vi "MyTest_maximumSequence.vi"() -> ()   [LabVIEW 2018]
uses:
  VisionLibrariesXimea/xiLib/xiLIB_64bit/xiLIB/xiCamLib/xiLIB/Typedefs/xiLIB - PRM_Type.ctl
  VisionLibrariesXimea/xiLib/xiLIB_64bit/xiLIB/xiCamLib/xiLIB/Typedefs/xiLIB - PRM_Function.ctl
  VisionLibrariesXimea/xiLib/xiLIB_64bit/xiLIB/xiCamLib/xiCam/PRM/PRM/PRM_v2.ctl
  VisionLibrariesXimea/xiLib/xiLIB_64bit/xiLIB/xiCamLib/xiCam/PRM/ACQ_TIMING_MODE/ACQ_TIMING_MODE.ctl
  VisionLibrariesXimea/xiLib/xiLIB_64bit/xiLIB/xiCamLib/xiLIB/xiLIB - GetPRM_INFO.vi
  VisionLibrariesXimea/xiLib/xiLIB_64bit/xiLIB/xiCamLib/xiCam/Methods/xiCam - GetParam_Int32.vi
  VisionLibrariesXimea/xiLib/xiLIB_64bit/xiLIB/xiCamLib/xiCam/Methods/xiCam - GetParam_Float.vi
  VisionLibrariesXimea/xiLib/xiLIB_64bit/xiLIB/xiCamLib/xiCam/Methods/xiCam - GetParam_String.vi
panel:
  out "VI running":i32
  in  "input PRM":T1=enum."IMAGE_DATA_FORMAT_RGB32_ALPHA"
  out "Method":T2
  out "Type":T3
  out "output":variant
  in  "ask":bool
  out "error out":errorcluster
  in  "tot frame number":i32=10
  in  "stop":bool
  out "FFT":dbl[][](graph)
  out "Intensity Graph":u8[][](graph)
  in  "Exposure (us)":i32(slide) caption="Exposure (us) 1us - 1s steps of 1us" min=1 max=1000000 scale=0.9..5000.0
  in  "Height":i32 min=2 max=3424
  in  "Width":i32 min=32 max=4704
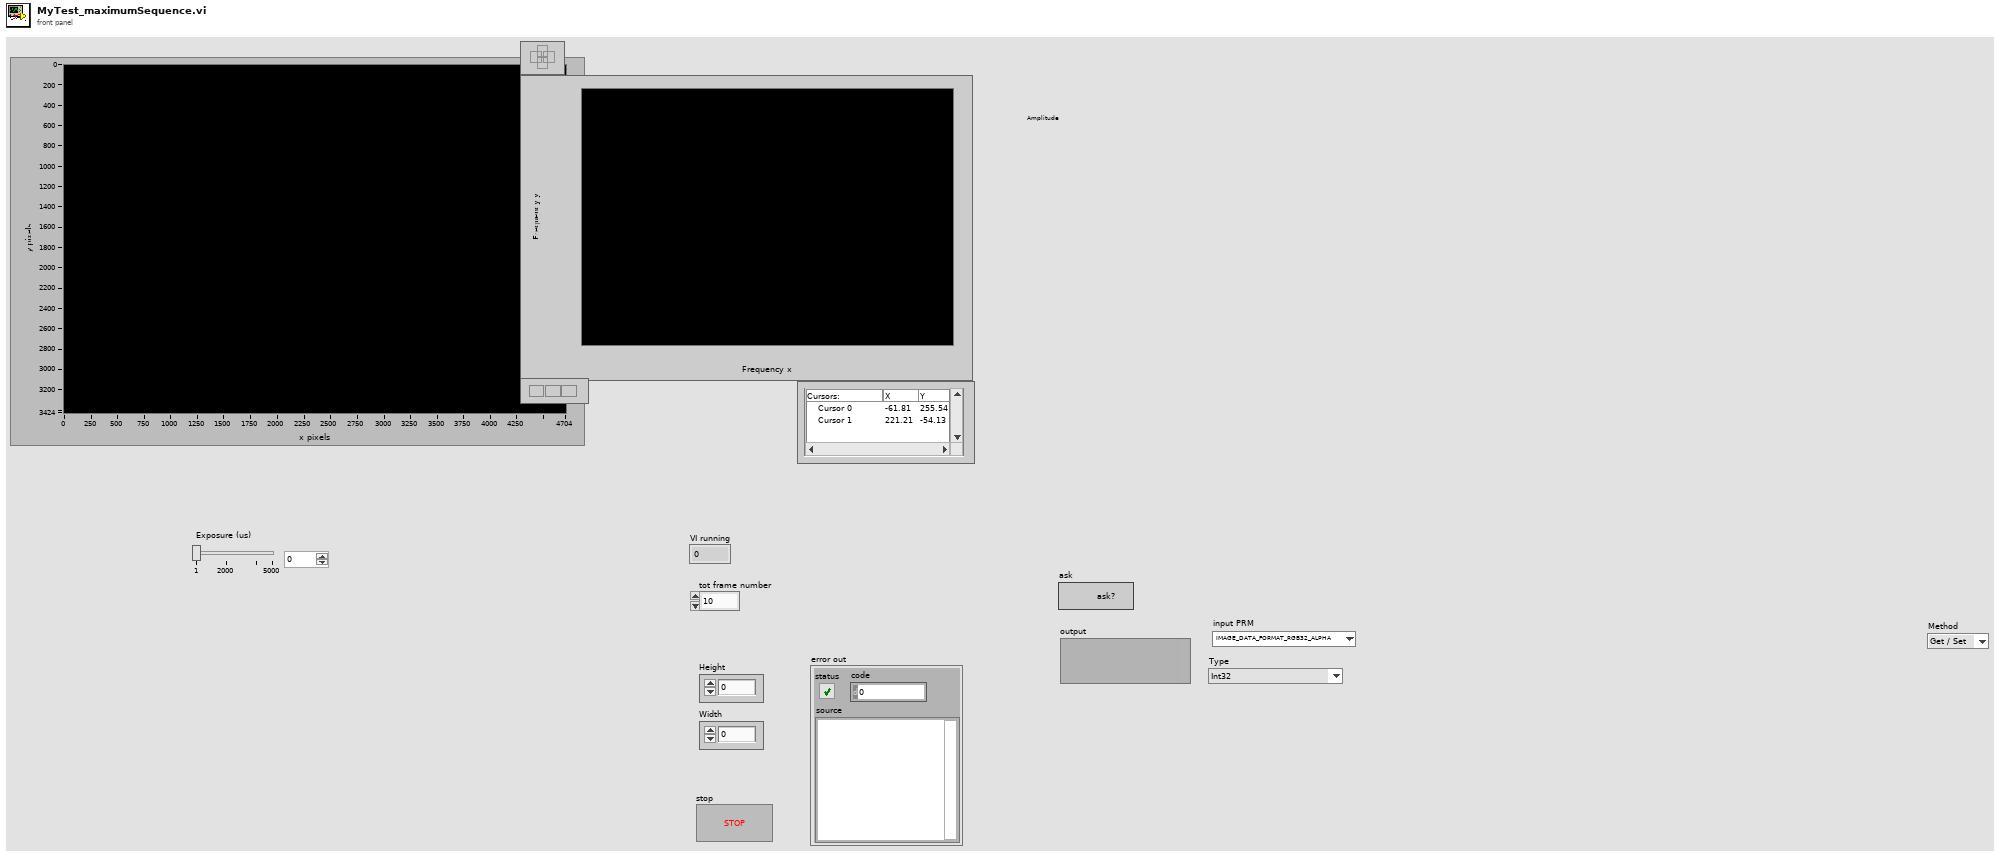
[diagram p1: front panel]
types:
  T1 = typedef "PRM_v2.ctl" = enum16{"ACQ_BUFFER_SIZE", "ACQ_FRAME_BURST_COUNT", "ACQ_TIMING_MODE", "ACQ_TRANSPORT_BUFFER_SIZE", "AE_MAX_LIMIT", "AEAG", "AEAG_LEVEL", "API_VERSION", "AG_MAX_LIMIT", "APPLY_CMS", "AUTO_BANDWIDTH_CALCULATION", "AUTO_WB", "AVAILABLE_BANDWIDTH", "AVAILABLE_BANDWIDTH_MAX", "AVAILABLE_BANDWIDTH_MIN", "BPC", "BUFFER_POLICY", "BUFFERS_QUEUE_SIZE", "CC_MATRIX_00", "CC_MATRIX_01", "CC_MATRIX_02", "CC_MATRIX_03", "CC_MATRIX_10", "CC_MATRIX_11", "CC_MATRIX_12", "CC_MATRIX_13", "CC_MATRIX_20", "CC_MATRIX_21", "CC_MATRIX_22", "CC_MATRIX_23", "CC_MATRIX_30", "CC_MATRIX_31", "CC_MATRIX_32", "CC_MATRIX_33", "CHIP_TEMP", "CMS", "COLOR_FILTER_ARRAY", "COOLING", "DEBOUNCE_EN", "DEBOUNCE_POL", "DEBOUNCE_T0", "DEBOUNCE_T1", "DEBUG_LEVEL", "DEFAULT_CC_MATRIX", "DEVICE_INSTANCE_PATH", "DEVICE_MODEL_ID", "DEVICE_NAME", "DEVICE_SN", "DEVICE_TYPE", "DEVICE_USER_ID", "DOWNSAMPLING", "DOWNSAMPLING_MAX", "DOWNSAMPLING_MIN", "DOWNSAMPLING_TYPE", "DRV_VERSION", "EXP_PRIORITY", "EXPOSURE", "EXPOSURE_DIRECT_UPDATE", "EXPOSURE_MAX", "EXPOSURE_MIN", "FFS_FILE_NAME", "FPGA1_VERSION", "FRAMERATE", "FRAMERATE_MAX", "FRAMERATE_MIN", "FREE_FFS_SIZE", "GAIN", "GAIN_DIRECT_UPDATE", "GAIN_MAX", "GAIN_MIN", "GAMMAC", "GAMMAY", "GPI_LEVEL", "GPI_MODE", "GPI_SELECTOR", "GPI_SELECTOR_MAX", "GPI_SELECTOR_MIN", "GPO_MODE", "GPO_SELECTOR", "GPO_SELECTOR_MAX", "GPO_SELECTOR_MIN", "HDR", "HDR_T1", "HDR_T2", "HEIGHT", "HEIGHT_MAX", "HEIGHT_MIN", "HOUSE_TEMP", "IMAGE_DATA_FORMAT", "IMAGE_IS_COLOR", "INPUT_CMS_PROFILE", "IS_COOLED", "IS_DEVICE_EXIST", "KNEEPOINT1", "KNEEPOINT2", "LED_MODE", "LED_SELECTOR", "LED_SELECTOR_MAX", "LED_SELECTOR_MIN", "LIMIT_BANDWIDTH", "LIMIT_BANDWIDTH_MAX", "LIMIT_BANDWIDTH_MIN", "LUT_EN", "LUT_INDEX", "LUT_INDEX_MAX", "LUT_INDEX_MIN", "LUT_VALUE", "LUT_VALUE_MAX", "LUT_VALUE_MIN", "MANUAL_WB", "MCU1_VERSION", "MCU2_VERSION", "OFFSET_X", "OFFSET_X_MAX", "OFFSET_X_MIN", "OFFSET_Y", "OFFSET_Y_MAX", "OFFSET_Y_MIN", "OUTPUT_CMS_PROFILE", "OUTPUT_DATA_BIT_DEPTH", "OUTPUT_DATA_PACKING", "READ_FILE_FFS", "RECENT_FRAME", "SENSOR_DATA_BIT_DEPTH", "SENSOR_MODE", "SENSOR_TAPS", "SHARPNESS", "SHUTTER_TYPE", "TARGET_TEMP", "TRG_DELAY", "TRG_SELECTOR", "TRG_SOFTWARE", "TRG_SOURCE", "USED_FFS_SIZE", "WB_KB", "WB_KG", "WB_KR", "WIDTH", "WIDTH_MAX", "WIDTH_MIN", "WRITE_FILE_FFS", "ACQ_BUFFER_SIZE_UNIT", "ACQ_TRANSPORT_BUFFER_COMMIT", "AEAG_ROI_HEIGHT", "AEAG_ROI_OFFSET_X", "AEAG_ROU_OFFSET_Y", "AEAG_ROI_WIDTH", "API_CONTEXT_LIST", "BINNING_HORIZONTAL", "BINNING_SELECTOR", "BINNING_VERTICAL", "COLUMN_FPN_CORRECTION", "COUNTER_SELECTOR", "COUNTER_VALUE", "DECIMATION_HORIZONTAL", "DECIMATION_SELECTOR", "DECIMATION_VERTICAL", "DEVICE_ID", "DEVICE_LOCATION_PATH", "DEVICE_MANIFEST", "DEVICE_RESET", "DEVICE_SENS_SN", "EXPOSURE_BURST_COUNT", "FFS_ACCESS_KEY", "GAIN_SELECTOR", "HW_REVISION", "IMAGE_BLACK_LEVEL", "IMAGE_DATA_BIT_DEPTH", "IMAGE_DATA_FORMAT_RGB32_ALPHA", "IMAGE_PAYLOAD_SIZE", "LENS_APERTURE_VALUE", "LENS_FEATURE", "LENS_FEATURE_SELECTOR", "LENS_FOCAL_LENGTH", "LENS_FOCUS_DISTANCE", "LENS_FOCUS_MOVE", "LENS_FOCUS_MOVEMENT_VALUE", "LENS_MODE", "OUTPUT_DATA_PACKING_TYPE", "SENSOR_CLOCK_FREQ_HZ", "SENSOR_CLOCK_FREQ_INDEX", "SENSOR_FEATURE_SELECTOR", "SENSOR_FEATURE_VALUE", "SENSOR_OUTPUT_CHANNEL_COUNT", "TRANSPORT_PIXEL_FORMAT", "TS_RST_MODE", "TS_RST_SOURCE"}
  T2 = typedef "xiLIB - PRM_Function.ctl" = enum16{"Get / Set", "Get", "Set"}
  T3 = typedef "xiLIB - PRM_Type.ctl" = enum16{"Int32", "Float", "String", "DOWNSAMPLING_TYPE", "IMAGE_DATA_FORMAT", "BUFFER_POLICY", "TRG_SOURCE", "GPI", "GPO", "ACQ_TIMING_MODE", "BINNING_PATTERN", "BINNING_SELECTOR", "CMS_MODE", "COUNTER_SELECTOR", "DEBUG_LEVEL", "DECIMATION_PATTERN", "DECIMATION_SELECTOR", "GAIN_SELECTOR_TYPE", "LED_MODE", "LENS_FEATURE_SELECTOR", "LENS_MODE", "OUTPUT_DATA_PACKING_TYPE", "SENSOR_FEATURE_SELECTOR", "SHUTTER_TYPE", "TRG_SELECTOR", "TS_RST_MODE", "TS_RST_SOURCE"}
  T4 = typedef "ACQ_TIMING_MODE.ctl" = enum16{"FREE_RUN", "FRAME_RATE"}
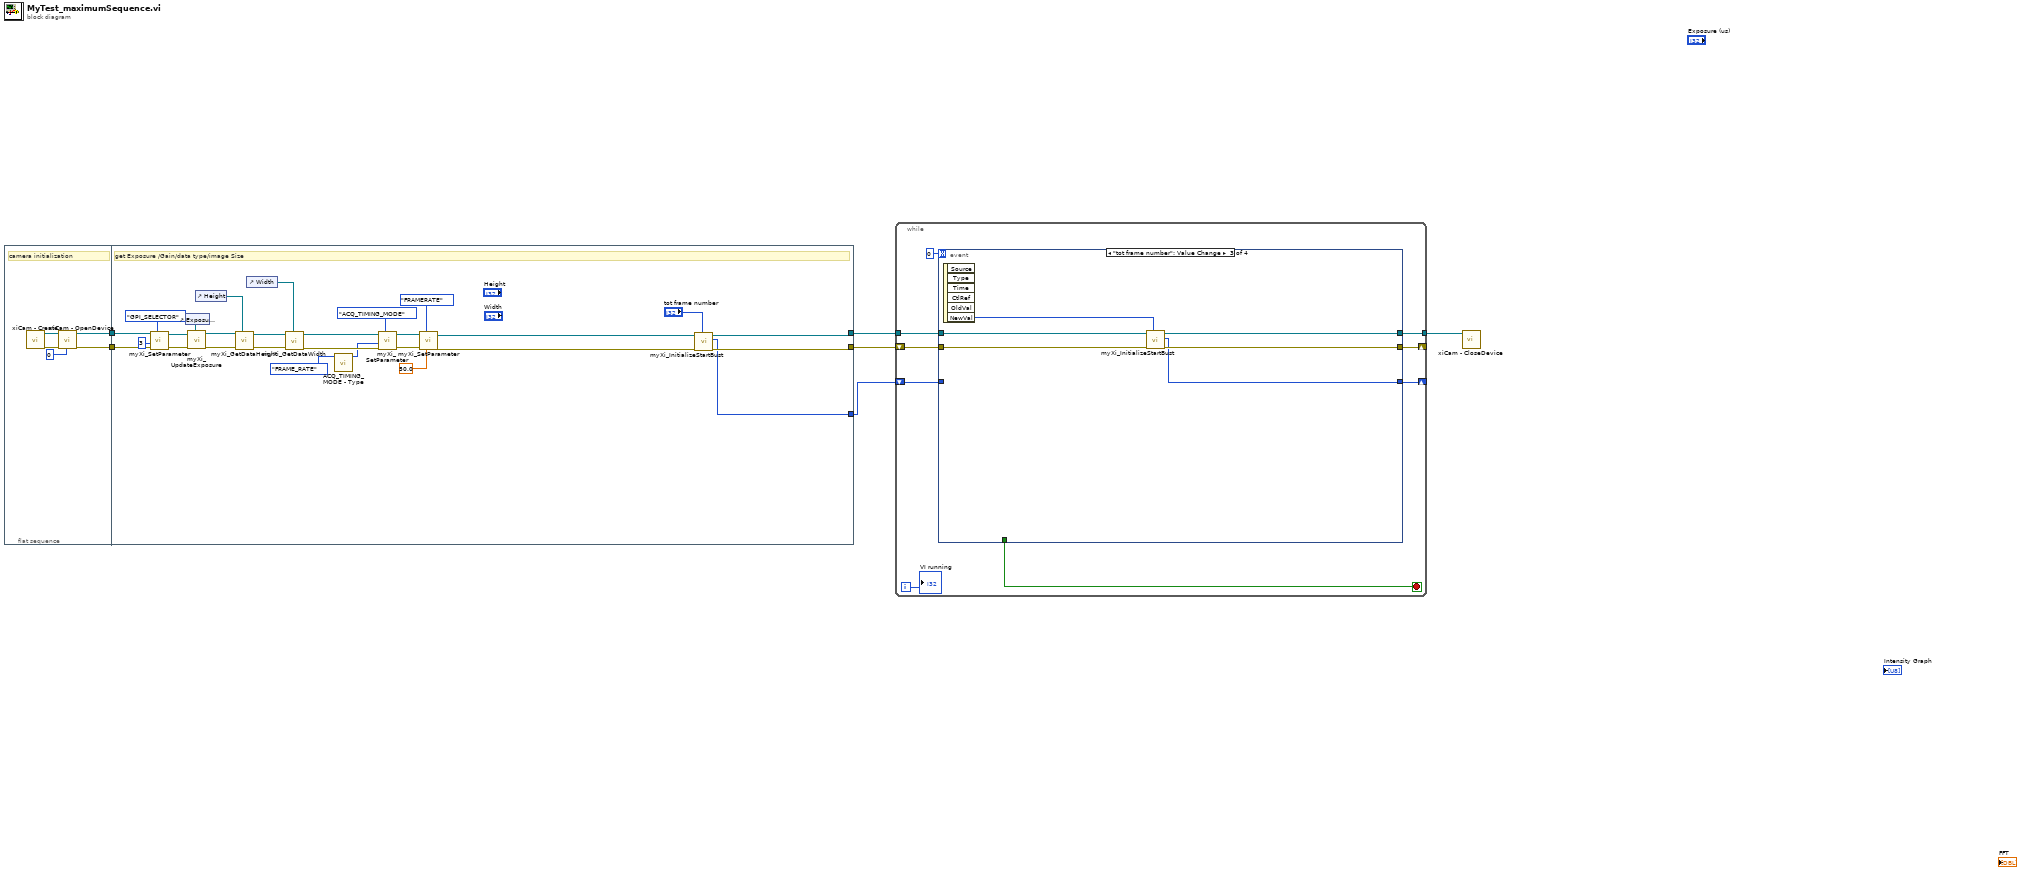
[diagram p0: block diagram]
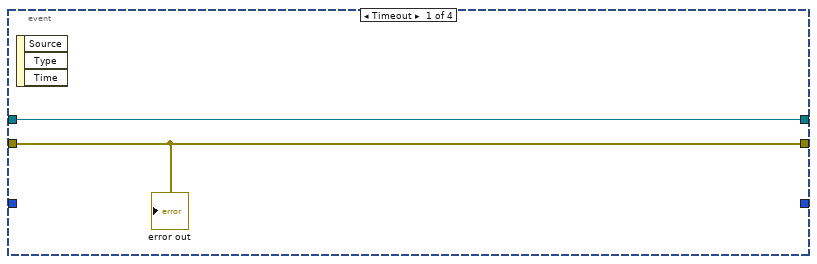
[diagram p2: hidden frame]
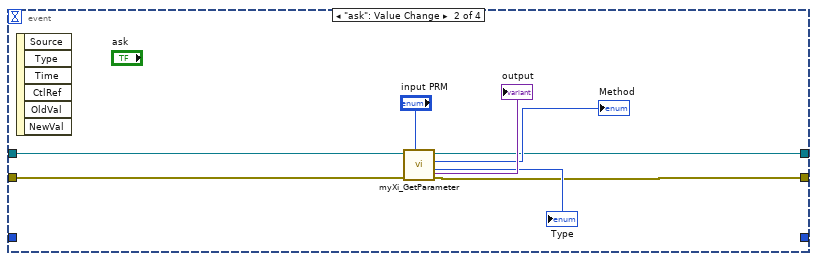
[diagram p3: hidden frame]
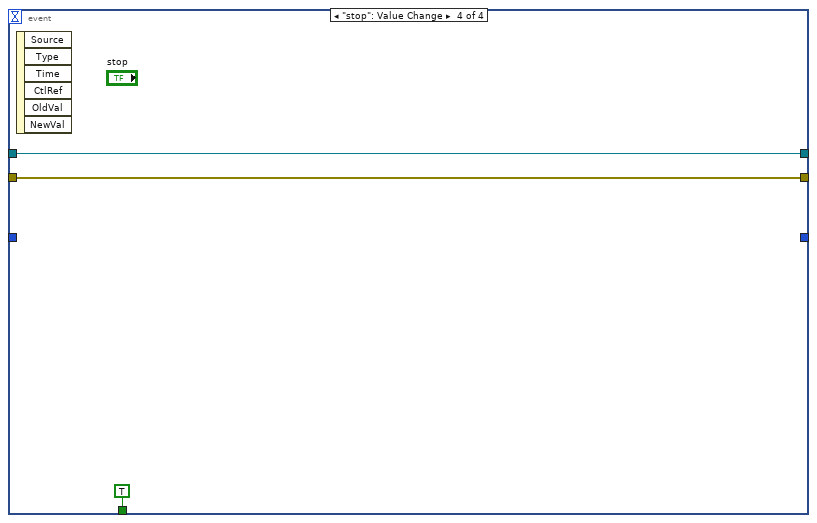
[diagram p4: hidden frame]
diagram:
  n1 = flat-sequence {
    tunnel: [w11] -> w6
    tunnel: [w10] -> w5
    tunnel: [w16] -> w3
    tunnel: [w14] -> w4
    tunnel: w6 -> [w30]
    tunnel: w5 -> [w32]
    tunnel: [w12] -> w1
    frame #0 {
      # "camera initialization"
      n2 = call "xiCam - Create.vi"() -> ("error out"=w8:errorcluster, "new xiCam"=w9:refnum<k24>)  [unwired: 10 in]
      n3 = call "xiCam - OpenDevice.vi"("DevID"=0, "error in (no error)"=w8, "xiCam In"=w9) -> ("error out"=w10:errorcluster, "xiCam Out"=w11:refnum<k24>)  [unwired: 7 in]
    }
    frame #1 {
      # "get Exposure /Gain/data type/image Size"
      n4 = call "myXi_SetParameter.vi"("input PRM"=PRM_v2."GPI_SELECTOR", "error in"=w32, "input value I32"=3, "xiCam IN"=w30) -> ("error out"=w31:errorcluster, "xiCam Out"=w29:refnum<k24>)  [unwired: 6 in]
      n5 = control-ref of="Exposure (us)"() -> (w39:refnum<vi>)
      n6 = call "myXi_UpdateExposure.vi"("Exposure (us)"=w39, "error in"=w31, "xiCam In"=w29) -> ("error out"=w37:errorcluster, "xiCam Out"=w38:refnum<k24>)  [unwired: 7 in]
      n7 = control-ref of="Height"() -> (w36:refnum<vi>)
      n8 = call "myXi_GetDataHeight.vi"("Height"=w36, "error in"=w37, "xiCam In"=w38) -> ("error out"=w34:errorcluster, "xiCam Out"=w35:refnum<k24>)  [unwired: 6 in, 1 out]
      n9 = control-ref of="Width"() -> (w33:refnum<vi>)
      n10 = call "myXi_GetDataWidth.vi"("width"=w33, "error in"=w34, "xiCam In"=w35) -> ("error out"=w25:errorcluster, "xiCam Out"=w26:refnum<k24>)  [unwired: 6 in, 1 out]
      n11 = call "ACQ_TIMING_MODE - Type.vi"("ACQ TIMING MODE"=ACQ_TIMING_MODE."FRAME_RATE") -> ("ACQ_TIMING_MODE_VALUE"=w22:i32)  [unwired: 9 in, 1 out]
      n12 = call "myXi_SetParameter.vi"("input PRM"=PRM_v2."ACQ_TIMING_MODE", "error in"=w25, "input value I32"=w22, "xiCam IN"=w26) -> ("error out"=w21:errorcluster, "xiCam Out"=w20:refnum<k24>)  [unwired: 6 in]
      n13 = call "myXi_SetParameter.vi"("input value DBL"=sgl 50.0, "input PRM"=PRM_v2."FRAMERATE", "error in"=w21, "xiCam IN"=w20) -> ("error out"=w17:errorcluster, "xiCam Out"=w15:refnum<k24>)  [unwired: 6 in]
      n14 = call "myXi_InitializeStartBust.vi"("burst count"="tot frame number", "error in (no error)"=w17, "xiCam IN"=w15) -> ("error out"=w16:errorcluster, "Array"=w12:u8[], "xiCam Out"=w14:refnum<k24>)  [unwired: 6 in]
    }
  }
  n15 = while {
    tunnel: w4 -> [w47]
    tunnel: [w44] -> w2
    shift-right: [w46] -> _
    shift-left: w3 -> [w45]
    shift-right: [w41] -> _
    shift-left: w1 -> [w43]
    i -> [w40]
    stop <- w48 stop-if-true
    n16 = event shown="[2] \"tot frame number\": Value Change" {
      selector: _ -> [_ _ _ _]
      dyn-events: _ -> [_ _ _ _]
      timeout: 0 -> [_ _ _ _]
      tunnel: [_ _ _ TRUE ("stop")] -> w48
      tunnel: w47 -> [w49 w54 w64 w65]
      tunnel: [w50 w52 w60 w66] -> w46
      tunnel: w45 -> [w50 w53 w63 w66]
      tunnel: [w49 w51 w61 w65] -> w44
      tunnel: w43 -> [_ _ _ _]
      tunnel: [_ _ w59 _] -> w41
      event Timeout {
        n17 = event-data() -> ()  [unwired: 1 in, 3 out]
        "error out" <- w50
      }
      event "ask": Value Change {
        n18 = event-data() -> ()  [unwired: 1 in, 6 out]
        n19 = call "myXi_GetParameter.vi"("input PRM"="input PRM", "error in"=w53, "xiCam IN"=w54) -> ("error out"=w52:errorcluster, "Type"=→"Type":T3, "Method"=→"Method":T2, "xiCam Out"=w51:refnum<k24>, "output"=→"output":variant)  [unwired: 3 in, 1 out]
      }
      event "tot frame number": Value Change {
        n20 = event-data() -> ("NewVal"=w62:i32)  [unwired: 1 in, 5 out]
        n21 = call "myXi_InitializeStartBust.vi"("burst count"=w62, "error in (no error)"=w63, "xiCam IN"=w64) -> ("error out"=w60:errorcluster, "Array"=w59:u8[], "xiCam Out"=w61:refnum<k24>)  [unwired: 6 in]
      }
      event "stop": Value Change {
        n22 = event-data() -> ()  [unwired: 1 in, 6 out]
      }
    }
    "VI running" <- w40
  }
  n23 = call "xiCam - CloseDevice.vi"("xiCam In"=w2) -> ()  [unwired: 10 in, 1 out]
